vi "读取校准数据配置文件.vi"(8 "error in (no error)":errorcluster caption="错误输入（无错误）") -> (0 "错误输出":errorcluster)   [LabVIEW 2016, in "斯坦道CODMn新电路板.lvlib"]
uses:
  <vilib>/Utility/xml.llb/Read From XML File(string).vi
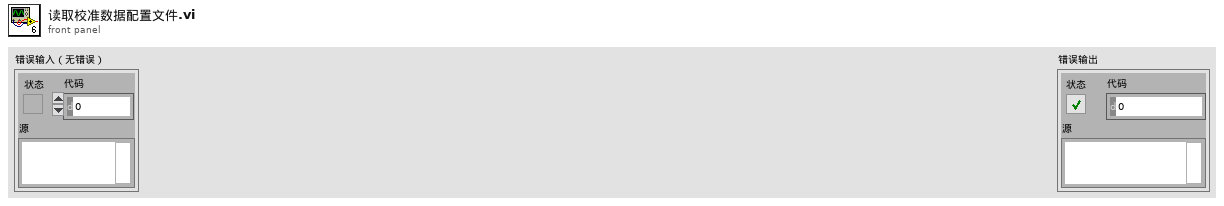
[diagram p1: front panel]
types:
  T1 = cluster{"CODMn曲线模型":cluster{"标液浓度1":dbl, "测量吸光度1":dbl, "样品1启用":bool, "标液浓度2":dbl, "测量吸光度2":dbl, "样品2启用":bool, "标液浓度3":dbl, "测量吸光度3":dbl, "样品3启用":bool, "标液浓度4":dbl, "测量吸光度4":dbl, "样品4启用":bool, "标液浓度5":dbl, "测量吸光度5":dbl, "样品5启用":bool, "模型":enum32{"线性", "多项式"}, "精度":dbl, "XY图":cluster{"X Values":dbl[], "Y Values":dbl[]}[], "拟合公式":string, "r^2":dbl, "标样一校准时间":timestamp, "标样二校准时间":timestamp, "标样三校准时间":timestamp, "标样四校准时间":timestamp, "标样五校准时间":timestamp, "二次方程":cluster{"c":dbl, "x":dbl, "x^2":dbl}, "标定时间":timestamp}[][]}
  T2 = cluster{"标液浓度1":dbl, "测量吸光度1":dbl, "样品1启用":bool, "标液浓度2":dbl, "测量吸光度2":dbl, "样品2启用":bool, "标液浓度3":dbl, "测量吸光度3":dbl, "样品3启用":bool, "标液浓度4":dbl, "测量吸光度4":dbl, "样品4启用":bool, "标液浓度5":dbl, "测量吸光度5":dbl, "样品5启用":bool, "模型":enum32{"线性", "多项式"}, "精度":dbl, "XY图":cluster{"X Values":dbl[], "Y Values":dbl[]}[], "拟合公式":string, "r^2":dbl, "标样一校准时间":timestamp, "标样二校准时间":timestamp, "标样三校准时间":timestamp, "标样四校准时间":timestamp, "标样五校准时间":timestamp, "二次方程":cluster{"c":dbl, "x":dbl, "x^2":dbl}, "标定时间":timestamp}[][]
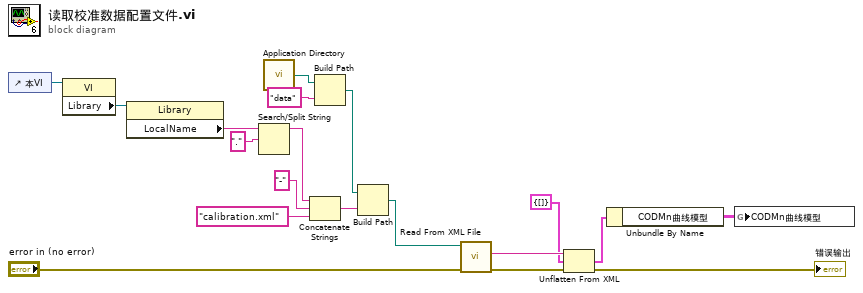
[diagram p0: block diagram]
diagram:
  n1 = control-ref of="本VI"() -> (w12:refnum<vi>)
  n2 = property class="VI"(reference=w12) -> ("Library"=w13:refnum<vi>)  [unwired: 1 in, 2 out]
  n3 = property class="Library"(reference=w13) -> ("LocalName"=w10:string)  [unwired: 1 in, 2 out]
  n4 = Search/Split String(string=w10, search string/char (-)="." ("搜索字符串/字符(-)")) -> (substring before match=w8:string)  [unwired: 1 in, 2 out]
  n5 = call <vilib>:"Application Directory.vi"() -> ("Application Directory"=w14:path)
  n6 = Concatenate Strings(w8, "-" ("字符串"), "calibration.xml" ("名称或相对路径")) -> (w5:string)
  n7 = Build Path(base path=w14, name or relative path="data" ("名称或相对路径")) -> (appended path=w11:path)
  n8 = Build Path(base path=w11, name or relative path=w5) -> (appended path=w4:path)
  n9 = call-poly <vilib>:"Read From XML File.vi"("error in (no error)"="error in (no error)", "XML File Path"=w4) -> ("error out"=w18:errorcluster, "XML Elements"=w19:string)  [unwired: 7 in, 1 out]
  n10 = Unflatten From XML(xml string=w19, type=T1 {"CODMn曲线模型"=[]} ("输出簇"), error in (no error)=w18) -> (value=w3:T1, error out=→"错误输出":errorcluster)
  n11 = Unbundle By Name(w3) -> ("CODMn曲线模型"=w1:T2)
  n12 = global write "校准数据全局变量.vi" "CODMn曲线模型"(w1) -> ()
